vi "Inverse_STFT.vi"(5 "Selected":i32[](array[numeric]), 6 "전체_Selected":i32[](array[numeric]), 7 "Group Number":i32, 10 "W":dbl[][](array[numeric]), 11 "STFT Spectrogram {X}":dbl[][](array[numeric])) -> (3 "Inverse_STFT":dbl[](array[numeric]))   [LabVIEW 2014]
uses:
  <vilib>/Analysis/baseanly.llb/Real A x B.vi
  <vilib>/Analysis/2dsp.llb/Inverse Real FFT.vi
  <vilib>/Analysis/Matrix/Numeric/Conversions/Matrix To Array - RM.vi
  <vilib>/Analysis/NI_AALBase.lvlib
  <vilib>/Analysis/Matrix/NI_Matrix.lvlib
  <vilib>/Analysis/NI_AALPro.lvlib
panel:
  out "transposed array":dbl[][](array[numeric])
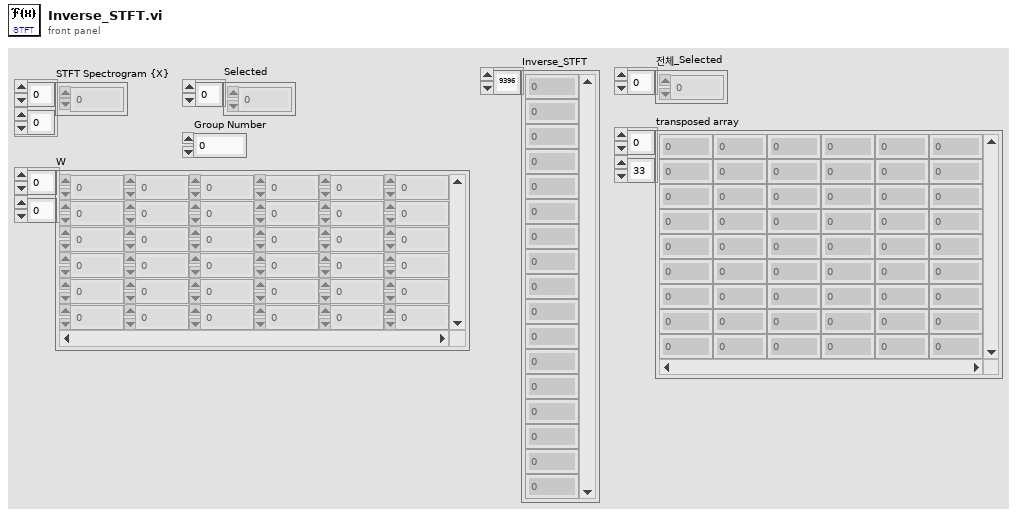
[diagram p1: front panel]
types:
  T1 = typedef "NI_Matrix.lvlib/RealMatrix.ctl" = dbl[][]
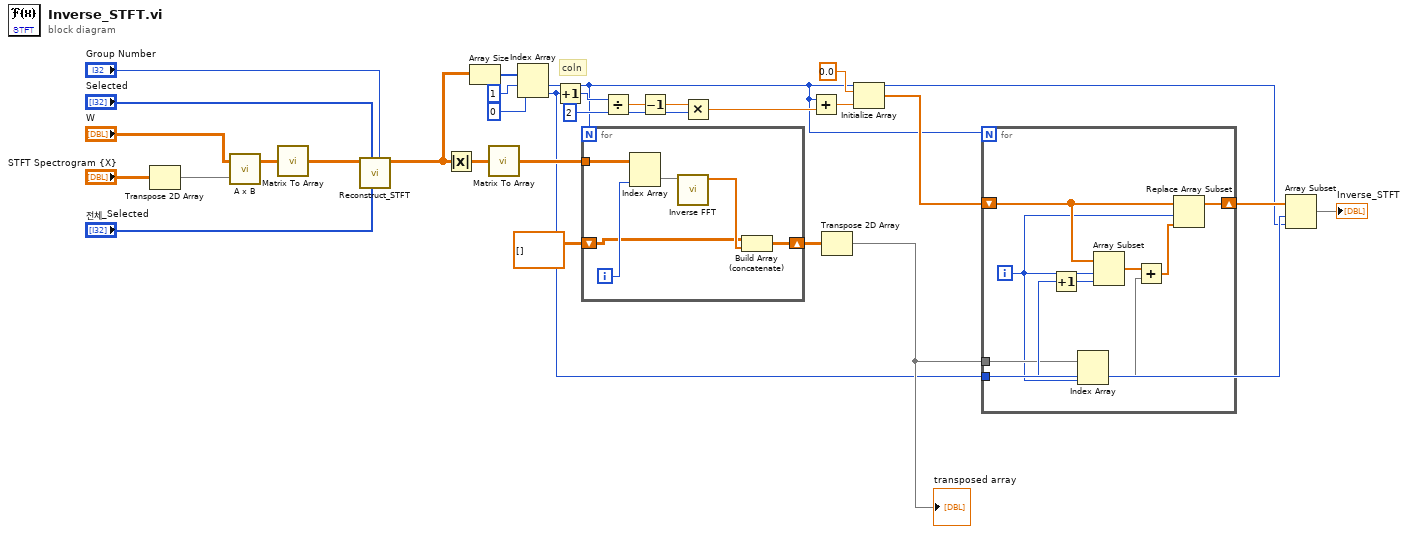
[diagram p0: block diagram]
diagram:
  w17 = 2 ("y")
  # "coln"
  n1 = Transpose 2D Array(2D array="STFT Spectrogram {X}") -> (transposed array=w29:dbl[][])
  n2 = call-poly <vilib>:"A x B.vi"("B"=w29, "A"="W") -> ("A x B"=w6:T1)  [unwired: 1 out]
  n3 = call-poly <vilib>:"Matrix To Array.vi"("Real Matrix"=w6) -> ("Real 2D Array"=w5:dbl[][])
  n4 = call "Reconstruct_STFT.vi"("Group Number"="Group Number", "전체_Selected"="전체_Selected", "Selected"="Selected", "STFT_CutOff"=w5) -> ("STFT_FULL"=w1:dbl[][])  [unwired: 7 in]
  n5 = Absolute Value ("Absolute Value.vi")(x=w1) -> (abs(x)=w7:dbl[][])
  n6 = Array Size(array=w1) -> (size(s)=w26:i32[])
  n7 = call-poly <vilib>:"Matrix To Array.vi"("Real Matrix"=w7) -> ("Real 2D Array"=w24:dbl[][])
  n8 = Index Array(array=w26, index #1=1 ("index"), index #2=0 ("index")) -> (element #1=w9:i32, element #2=w10:i32)
  n9 = Increment(x=w10) -> (x+1=w20:i32)
  n10 = for {
    N: w9 -> [_]
    tunnel: w24 -> [w35]
    shift-right: [w31] -> w22
    shift-left: dbl[][] [] -> [w30]
    i -> [w34]
    n11 = Index Array(array=w35, index (col)=w34) -> (element=w33:dbl[])  [unwired: 1 in]
    n12 = call-poly <vilib>:"Inverse FFT.vi"("FFT {X}"=w33) -> ("X"=w32:dbl[])  [unwired: 9 in, 1 out]
    n13 = Build Array (concatenate)(w30, w32) -> (w31:dbl[][])
  }
  n14 = Divide(x=w20, y=w17) -> (x/y=w19:dbl)
  n15 = Decrement(x=w19) -> (x-1=w18:dbl)
  n16 = Multiply(x=w18, y=w17) -> (x*y=w16:dbl)
  n17 = Add(x=w9, y=w16) -> (x+y=w15:dbl)
  n18 = Transpose 2D Array(2D array=w22) -> (transposed array=w21:dbl[][])
  "transposed array" <- w21
  n19 = Initialize Array(0.0 ("element"), w15) -> (w13:dbl[])
  n20 = for {
    N: w9 -> [_]
    tunnel: w21 -> [w41]
    shift-right: [w36] -> w11
    shift-left: w13 -> [w44]
    tunnel: w10 -> [w43]
    i -> [w37]
    n21 = Increment(x=w43) -> (x+1=w42:i32)
    n22 = Index Array(array=w41, index (col)=w37) -> (element=w39:dbl[])  [unwired: 1 in]
    n23 = Array Subset(array=w44, index=w37, length=w42) -> (w40:dbl[])
    n24 = Add(x=w40, y=w39) -> (x+y=w38:dbl[])
    n25 = Replace Array Subset(array=w44, new element=w38, index=w37) -> (w36:dbl[])
  }
  n26 = Array Subset(array=w11, index=w10, length=w9) -> (→"Inverse_STFT":dbl[])
